vi "TabConAlt v0.1.vi"() -> ()   [LabVIEW 2017]
panel:
  out "strMAT":string
  in  "initMAT":bool
  out "statusMAT":bool
  out "connMAT":bool caption="Matisse TX"
  out "strMIL":string
  in  "initMIL":bool
  out "statusMIL":bool
  out "connMIL":bool caption="Millenia eV 25W"
  out "strCCD":string
  in  "initCCD":bool
  out "statusCCD":bool
  out "connCCD":bool caption="Pylon CCD"
  out "strSPT":string
  in  "initSPT":bool caption="Spectrometer"
  out "statusSPT":bool
  out "connSPT":bool caption="Spectrometer"
  out "strLIA":string
  in  "initLIA":bool caption="Lock-in"
  out "statusLIA":bool
  out "connLIA":bool caption="Lock-in & Chopper"
  in  "initALL":bool caption="Initialize all"
  in  "stopExecution":bool
  in  "clearNotifications":bool
  out "Notifications":string
  out "measRUN":bool caption="Measurement running"
  out "measREADY":bool caption="Measurement ready"
  out "UIbusy":bool caption="Interface busy"
  in  "Settings":T1(tab)
  in  "visaSPT":string caption="VISA address"
  in  "visaCCD":string caption="VISA address"
  in  "visaLIA":string caption="VISA address"
  in  "Chopping Frequency":dbl[unit](knob) scale=200.0..2000.0
  in  "Ring cavity  energy":cluster{dbl[unit], dbl[unit]}(slide) caption="Ring cavity  energy / eV"
  in  "Ring cavity wavelength":cluster{dbl[unit], dbl[unit]}(slide)={0.0, 9.616279069767442e-07} caption="Ring cavity wavelength / nm"
  in  "Enslave Millennia eV":bool
  in  "Installed Optics":string(combo)="MOS2 BB"
  in  "visaMAT":string caption="VISA address"
  in  "Matisse Power":dbl[unit](knob)=1e-06 caption="Millenia Power" min=1.0 max=25.0 scale=1.0..25.0
  in  "visaMIL":string caption="VISA address"
  in  "Millenia Power":dbl[unit](knob)=0.001 min=1.0 max=25.0 scale=1.0..25.0
  out "DummyVisaOut":string
  in  "mainqSize":dbl=1000.0 caption="Queue size" min=1.0 step=1.0
  in  "timebaseMaster":dbl[unit]=0.08 caption="Master timebase" min=0.0001 max=0.5 step=0.0001 format="%#_6f"
  in  "timebaseSlave":dbl[unit]=0.16 caption="Slave timebase" min=0.0001 max=0.5 step=0.0001
  in  "abbrSPT":string="SPT"
  in  "abbrCCD":string="CCD"
  in  "abbrMIL":string="MIL"
  in  "abbrMAT":string="MAT"
  in  "abbrLIA":string="LIA"
  in  "nameSPT":string="Spectrometer"
  in  "nameLIA":string="SRS865"
  in  "nameCCD":string="Pylon CCD"
  in  "nameMIL":string="Millennia eV 25W"
  in  "nameMAT":string="Matisse 2 TX"
  # "Lower"
  # "Upper"
  # "eV"
  # "eV"
  # "Lower"
  # "Upper"
  # "nm"
  # "nm"
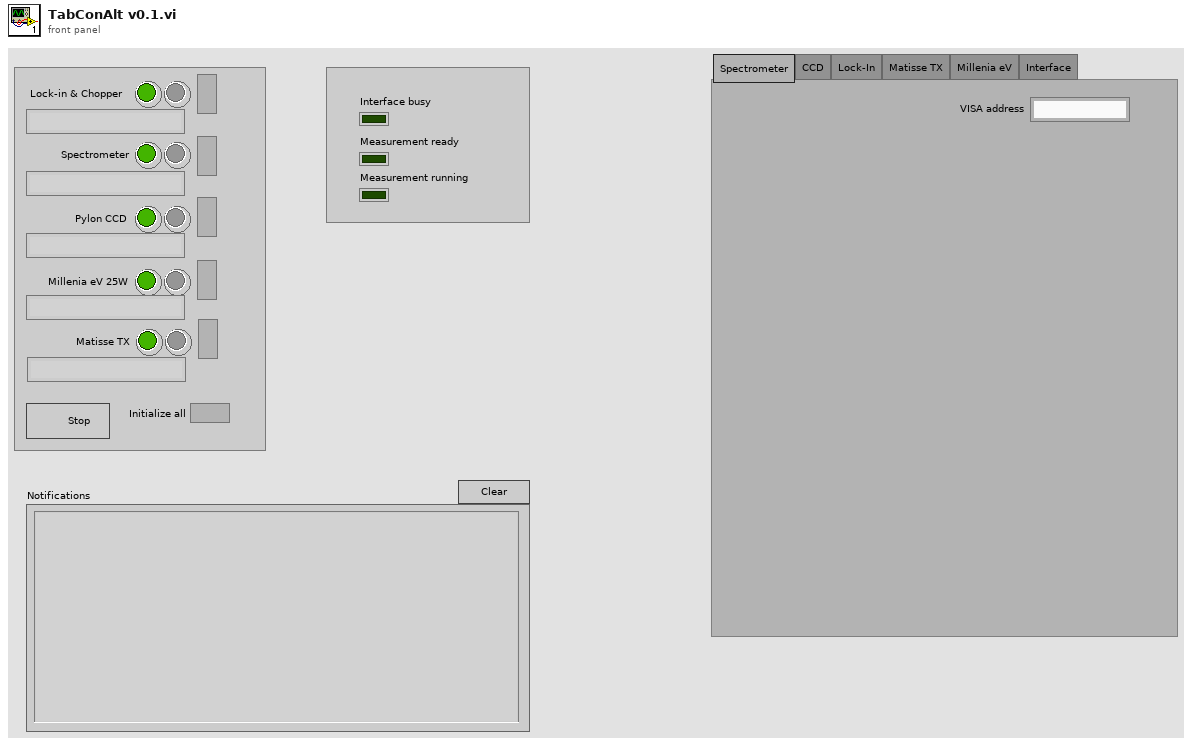
[diagram p1: front panel]
types:
  T1 = enum32{"Spectrometer", "CCD", "Lock-In", "Matisse TX", "Millenia eV", "Interface"}
  T2 = cluster{"elementArr":cluster{"cmd":string, "cmdclass":string, "data":variant}[]}
  T3 = cluster{"str":string, "ctlref":refnum<vi>, "newStatus":bool, "ctlstr":refnum<vi>}
  T4 = cluster{string, "chgStatusLED":refnum<user-event>}
  T5 = cluster{cluster{string, "chgStatusLED":refnum<user-event>}, cluster{string, "qintoMain":refnum<user-event>}}
  T6 = typedef "RefArray.ctl" = cluster{"String":string, "Array":refnum<vi>[]}[]
  T7 = cluster{"Command":string, "Command class":string, "Variant":variant}
  T8 = cluster{"Command":string, "Command class":string, "Variant":variant}[]
  T9 = cluster{"cmd":string, "cmdclass":string, "data":variant}[]
  T10 = typedef "eventsource.ctl" = u32
  T11 = cluster{"String":string, "String 2":string, "Variant":variant}[]
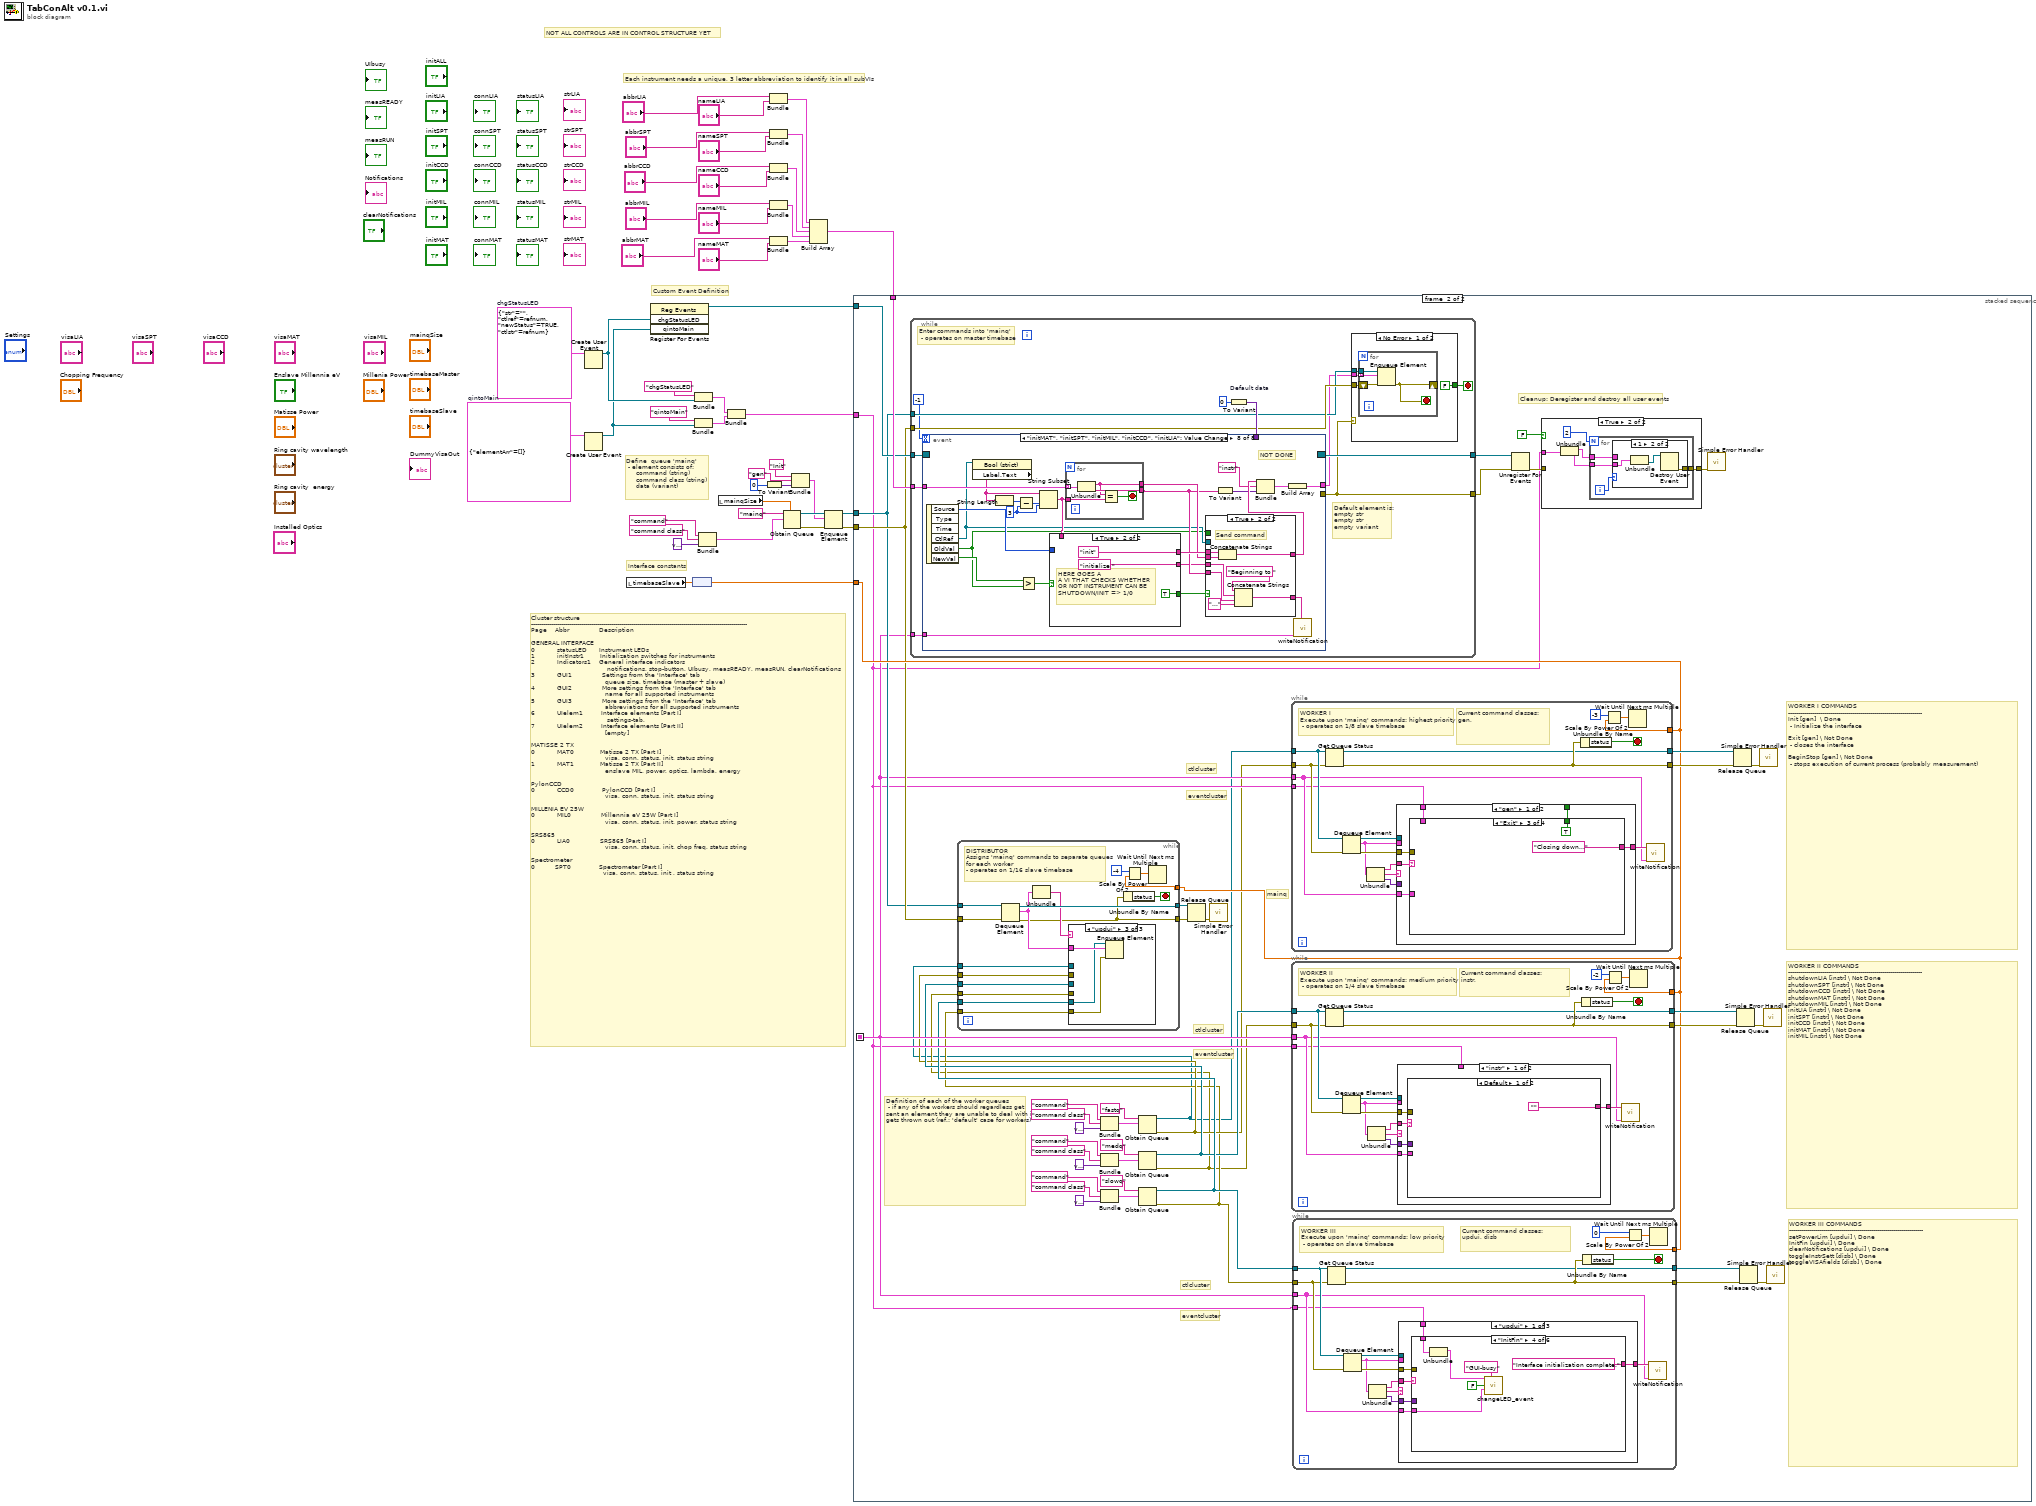
[diagram p0: block diagram]
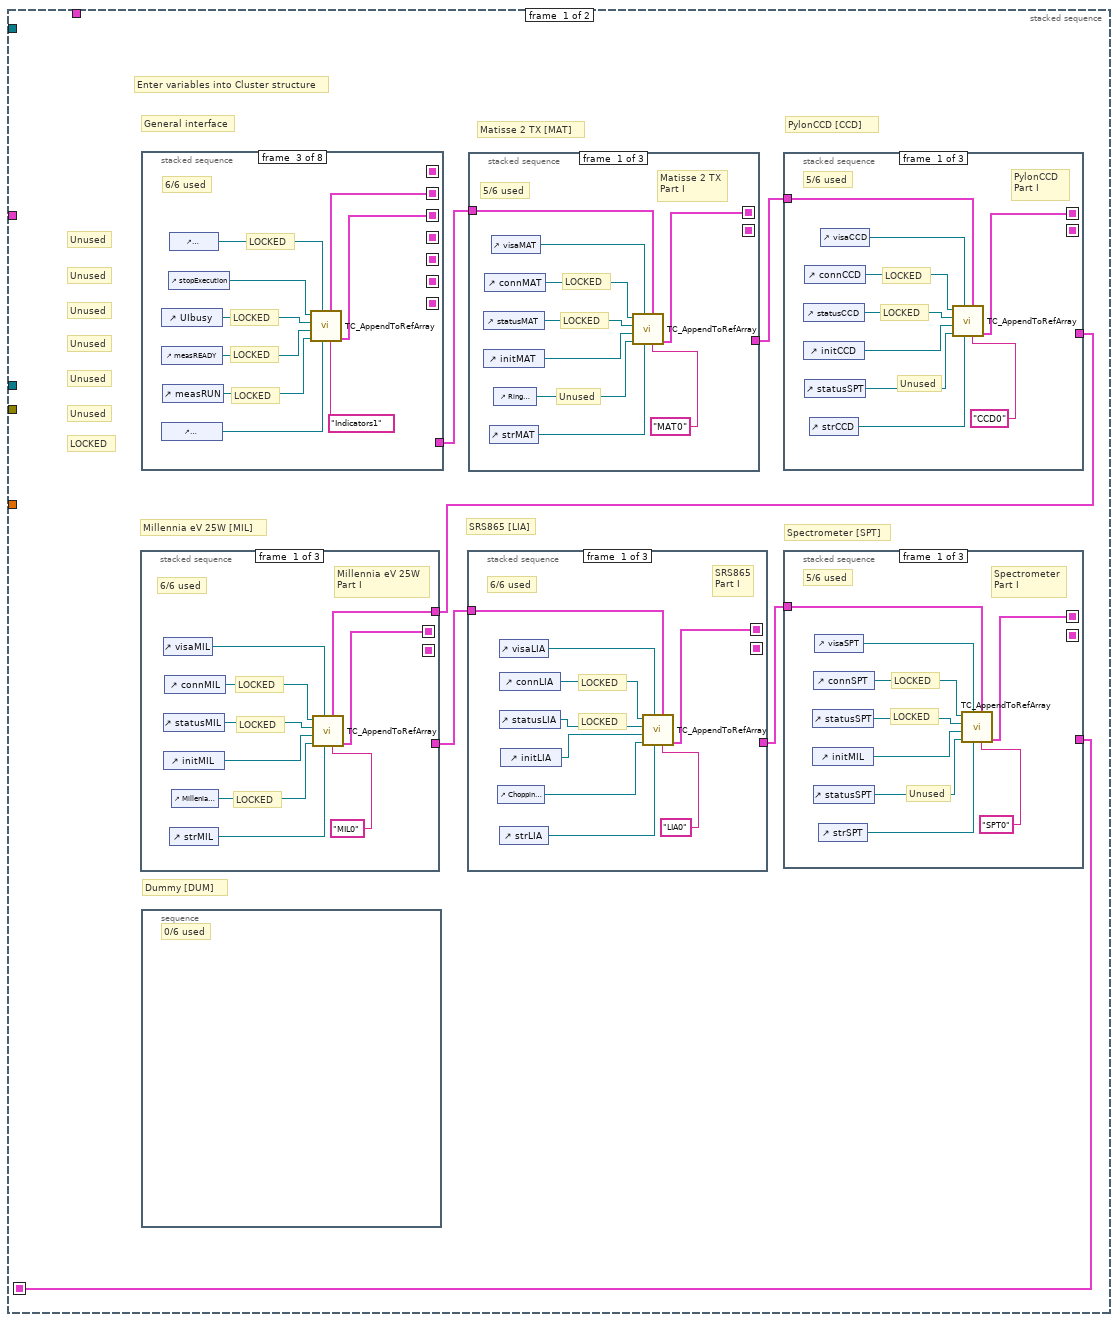
[diagram p2: hidden frame]
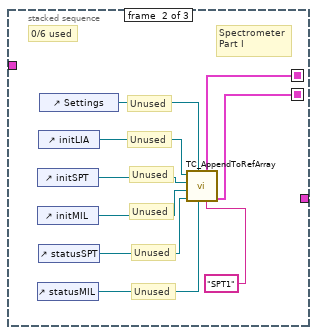
[diagram p3: hidden frame]
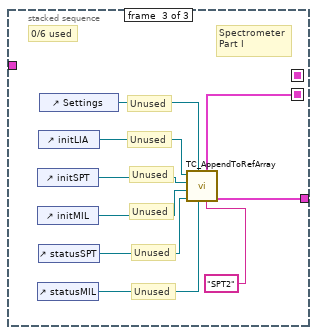
[diagram p4: hidden frame]
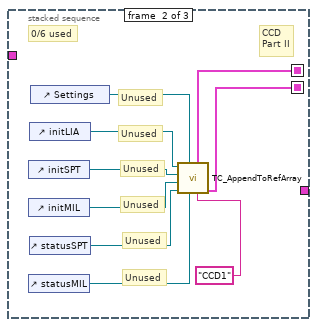
[diagram p5: hidden frame]
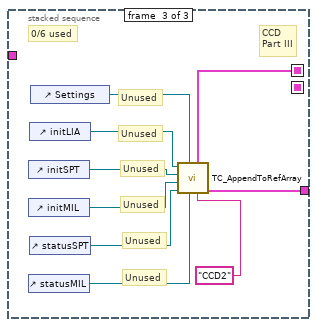
[diagram p6: hidden frame]
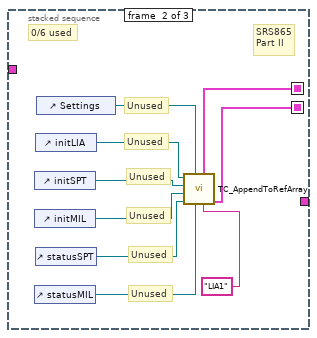
[diagram p7: hidden frame]
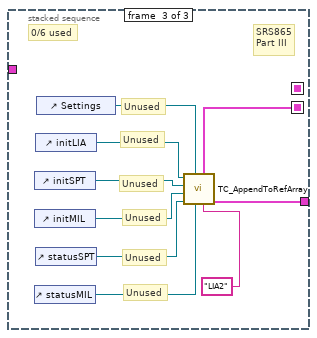
[diagram p8: hidden frame]
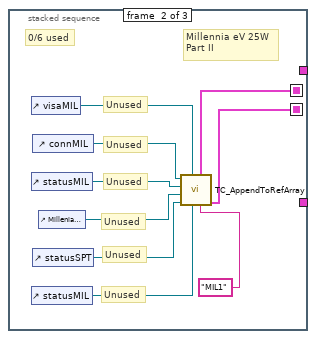
[diagram p9: hidden frame]
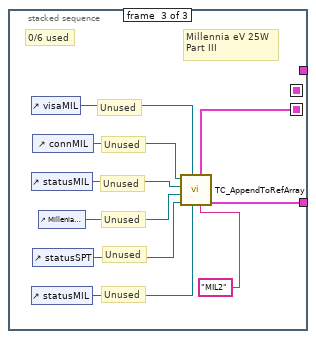
[diagram p10: hidden frame]
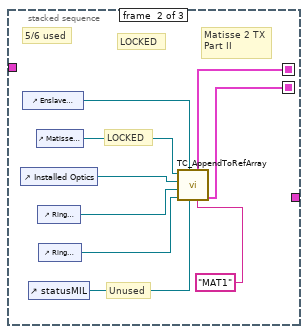
[diagram p11: hidden frame]
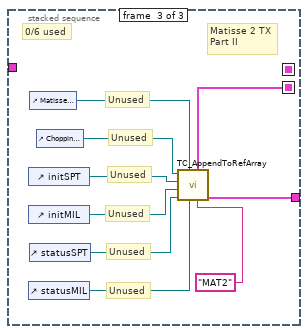
[diagram p12: hidden frame]
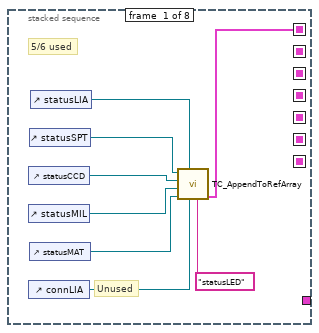
[diagram p13: hidden frame]
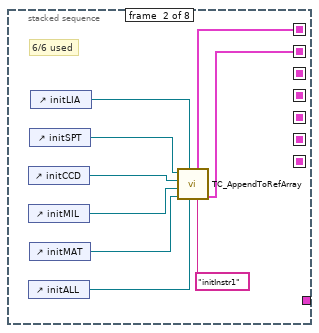
[diagram p14: hidden frame]
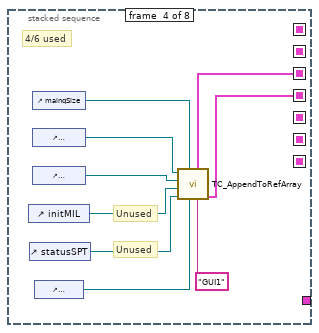
[diagram p15: hidden frame]
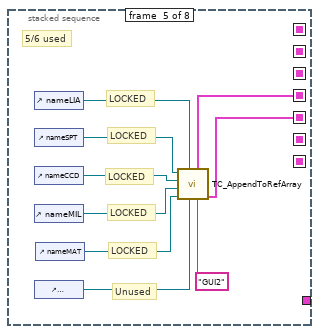
[diagram p16: hidden frame]
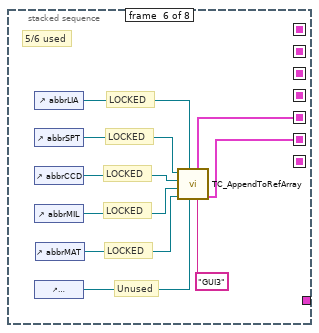
[diagram p17: hidden frame]
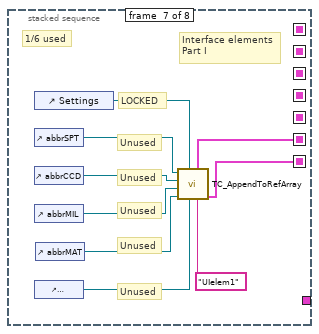
[diagram p18: hidden frame]
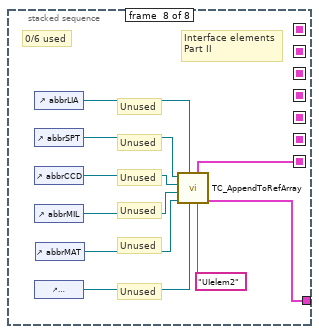
[diagram p19: hidden frame]
diagram:
  w13 = T2 {"elementArr"=[]}  # qintoMain
  w14 = T3 {"str"="", "ctlref"=refnum, "newStatus"=TRUE, "ctlstr"=refnum}  # chgStatusLED
  # "Custom Event Definition"
  # "Cluster structure\n------------------------------------------------------------------------------------------------------------\nPage    Abbr               Description\n\nGENERAL INTERFACE\n0           statusLED      Instrument LEDs\n1           initInstr1        Initialization switches for instruments\n2           Indicators1    General interface indicators\n                                      notifications, stop-button, UIbusy, measREADY, measRUN, clearNotifications\n3           GUI1               Settings from the 'Interface' tab\n                                     queue size, timebase (master + slave)\n4           GUI2               More settings from the 'Interface' tab\n                                     name for all supported instruments\n5           GUI3               More settings from the 'Interface' tab\n                                     abbreviations for all supported instruments\n6           UIelem1         Interface elements [Part I]\n                                      settings-tab,\n7           UIelem2         Interface elements [Part II]\n                                     [empty]\n\nMATISSE 2 TX\n0           MAT0             Matisse 2 TX [Part I]\n                                     visa, conn, status, init, status string\n1           MAT1             Matisse 2 TX [Part II]\n                                     enslave MIL, power, optics, lambda, energy\n\nPylonCCD\n0           CCD0              PylonCCD [Part I]\n                                     visa, conn, status, init, status string\n\nMILLENIA EV 25W\n0           MIL0               Millennia eV 25W [Part I]\n                                     visa, conn, status, init, power, status string\n\nSRS865\n0           LIA0               SRS865 [Part I]\n                                     visa, conn, status, init, chop freq, status string\n\nSpectrometer\n0          SPT0              Spectrometer [Part I]\n                                    visa, conn, status, init , status string"
  # "NOT ALL CONTROLS ARE IN CONTROL STRUCTURE YET"
  # "Each instrument needs a unique, 3 letter abbreviation to identify it in all subVIs"
  # "Define  queue 'mainq'\n - element consists of:\n     command (string)\n     command class (string)\n     data (variant)"
  # "Interface constants"
  n1 = Create User Event(user event datatype=w14) -> (user event=w12:refnum<user-event>)  [unwired: 1 in, 1 out]
  n2 = Create User Event(user event datatype=w13) -> (user event=w9:refnum<user-event>)  [unwired: 1 in, 1 out]
  n3 = local read "timebaseSlave"() -> (w33:dbl[unit])
  n4 = register-events(w12, w9) -> (reference out=w15:refnum<event-registration>)  [unwired: 2 in, 1 out]
  n5 = node(w33) -> (w32:dbl)
  n6 = Bundle("qintoMain", "qintoMain"=w9) -> (w2:cluster{string, "qintoMain":refnum<user-event>})  [unwired: 1 in]
  n7 = Bundle("chgStatusLED", "chgStatusLED"=w12) -> (w3:T4)  [unwired: 1 in]
  n8 = Bundle("command", "command class", variant) -> (w34:cluster{string, string, variant})  [unwired: 1 in]
  n9 = local read "mainqSize"() -> (w40:dbl)
  n10 = Bundle(w3, w2) -> (w1:T5)  [unwired: 1 in]
  n11 = To Variant(anything=0) -> (Variant=w42:variant)
  n12 = Bundle("abbrLIA"="abbrLIA", "nameLIA"="nameLIA") -> (w17:cluster{"abbrLIA":string, "nameLIA":string})  [unwired: 1 in]
  n13 = Bundle("abbrSPT"="abbrSPT", "nameSPT"="nameSPT") -> (w18:cluster{"abbrSPT":string, "nameSPT":string})  [unwired: 1 in]
  n14 = Bundle("abbrCCD"="abbrCCD", "nameCCD"="nameCCD") -> (w19:cluster{"abbrCCD":string, "nameCCD":string})  [unwired: 1 in]
  n15 = Bundle("abbrMIL"="abbrMIL", "nameMIL"="nameMIL") -> (w20:cluster{"abbrMIL":string, "nameMIL":string})  [unwired: 1 in]
  n16 = Bundle("abbrMAT"="abbrMAT", "nameMAT"="nameMAT") -> (w21:cluster{"abbrMAT":string, "nameMAT":string})  [unwired: 1 in]
  n17 = Obtain Queue(max queue size (-1, unlimited)=w40, name (unnamed)="mainq", element data type=w34) -> (queue out=w5:refnum<queue>, error out=w6:errorcluster)  [unwired: 2 in, 1 out]
  n18 = Bundle("Init", "gen", "Variant"=w42) -> (w4:cluster{string, string, "Variant":variant})  [unwired: 1 in]
  n19 = Build Array(w17, w18, w19, w20, w21) -> (w16:cluster{"abbrMAT":string, "nameMAT":string}[])
  n20 = Enqueue Element(queue=w5, element=w4, error in (no error)=w6) -> (queue out=w8:refnum<queue>, error out=w7:errorcluster)  [unwired: 1 in, 1 out]
  n21 = stacked-sequence {
    seq-local: [w44 _] -> [_ w263]
    tunnel: w32 -> [_ w275]
    tunnel: w16 -> [_ w273]
    tunnel: w15 -> [_ w269]
    tunnel: w1 -> [_ w262]
    tunnel: w8 -> [_ w264]
    tunnel: w7 -> [_ w265]
    frame #0 {
      # "LOCKED"
      # "Dummy [DUM]"
      # "Spectrometer [SPT]"
      # "PylonCCD [CCD]"
      # "Unused"
      # "Unused"
      # "Unused"
      # "Unused"
      # "Unused"
      # "Unused"
      # "SRS865 [LIA]"
      # "Millennia eV 25W [MIL]"
      # "General interface"
      # "Matisse 2 TX [MAT]"
      # "Enter variables into Cluster structure"
      n22 = stacked-sequence {
        seq-local: [w185 _ _ _ _ _ _ _] -> [_ w193 _ _ _ _ _ _]
        seq-local: [_ w194 _ _ _ _ _ _] -> [_ _ w204 _ _ _ _ _]
        seq-local: [_ _ w203 _ _ _ _ _] -> [_ _ _ w212 _ _ _ _]
        seq-local: [_ _ _ w211 _ _ _ _] -> [_ _ _ _ w221 _ _ _]
        seq-local: [_ _ _ _ w220 _ _ _] -> [_ _ _ _ _ w230 _ _]
        seq-local: [_ _ _ _ _ w229 _ _] -> [_ _ _ _ _ _ w239 _]
        seq-local: [_ _ _ _ _ _ w238 _] -> [_ _ _ _ _ _ _ w248]
        tunnel: [_ _ _ _ _ _ _ w247] -> w45
        frame #0 {
          # "Unused"
          # "5/6 used"
          n23 = control-ref of="statusCCD"() -> (w190:refnum<vi>)
          n24 = control-ref of="statusMIL"() -> (w189:refnum<vi>)
          n25 = control-ref of="connLIA"() -> (w187:refnum<vi>)
          n26 = control-ref of="statusSPT"() -> (w191:refnum<vi>)
          n27 = control-ref of="statusMAT"() -> (w188:refnum<vi>)
          n28 = control-ref of="statusLIA"() -> (w192:refnum<vi>)
          n29 = call "TC_AppendToRefArray.vi"("name"="statusLED", "ref6"=w187, "ref1"=w192, "ref5"=w188, "ref4"=w189, "ref3"=w190, "ref2"=w191) -> ("arrayOut"=w185:T6)  [unwired: 4 in]
        }
        frame #1 {
          # "6/6 used"
          n30 = control-ref of="initCCD"() -> (w199:refnum<vi>)
          n31 = control-ref of="initMIL"() -> (w198:refnum<vi>)
          n32 = control-ref of="initALL"() -> (w196:refnum<vi>)
          n33 = control-ref of="initSPT"() -> (w200:refnum<vi>)
          n34 = control-ref of="initMAT"() -> (w197:refnum<vi>)
          n35 = control-ref of="initLIA"() -> (w201:refnum<vi>)
          n36 = call "TC_AppendToRefArray.vi"("name"="initInstr1", "arrayIn"=w193, "ref6"=w196, "ref1"=w201, "ref5"=w197, "ref4"=w198, "ref3"=w199, "ref2"=w200) -> ("arrayOut"=w194:T6)  [unwired: 3 in]
        }
        frame #2 {
          # "LOCKED"
          # "LOCKED"
          # "LOCKED"
          # "LOCKED"
          # "6/6 used"
          n37 = control-ref of="UIbusy"() -> (w209:refnum<vi>)
          n38 = control-ref of="measREADY"() -> (w208:refnum<vi>)
          n39 = control-ref of="clearNotifications"() -> (w206:refnum<vi>)
          n40 = control-ref of="measRUN"() -> (w207:refnum<vi>)
          n41 = control-ref of="stopExecution"() -> (w202:refnum<vi>)
          n42 = control-ref of="Notifications"() -> (w210:refnum<vi>)
          n43 = call "TC_AppendToRefArray.vi"("name"="Indicators1", "arrayIn"=w204, "ref6"=w206, "ref1"=w210, "ref5"=w207, "ref4"=w208, "ref3"=w209, "ref2"=w202) -> ("arrayOut"=w203:T6)  [unwired: 3 in]
        }
        frame #3 {
          # "Unused"
          # "Unused"
          # "4/6 used"
          n44 = control-ref of="initMIL"() -> (w216:refnum<vi>)
          n45 = control-ref of="statusSPT"() -> (w215:refnum<vi>)
          n46 = control-ref of="mainqSize"() -> (w219:refnum<vi>)
          n47 = control-ref of="timebaseMaster"() -> (w218:refnum<vi>)
          n48 = control-ref of="timebaseSlave"() -> (w217:refnum<vi>)
          n49 = control-ref of="DummyVisaOut"() -> (w214:refnum<vi>)
          n50 = call "TC_AppendToRefArray.vi"("name"="GUI1", "arrayIn"=w212, "ref6"=w214, "ref1"=w219, "ref5"=w215, "ref4"=w216, "ref3"=w217, "ref2"=w218) -> ("arrayOut"=w211:T6)  [unwired: 3 in]
        }
        frame #4 {
          # "LOCKED"
          # "LOCKED"
          # "LOCKED"
          # "LOCKED"
          # "LOCKED"
          # "Unused"
          # "5/6 used"
          n51 = control-ref of="nameLIA"() -> (w228:refnum<vi>)
          n52 = control-ref of="nameSPT"() -> (w227:refnum<vi>)
          n53 = control-ref of="nameCCD"() -> (w226:refnum<vi>)
          n54 = control-ref of="nameMIL"() -> (w225:refnum<vi>)
          n55 = control-ref of="DummyVisaOut"() -> (w223:refnum<vi>)
          n56 = control-ref of="nameMAT"() -> (w224:refnum<vi>)
          n57 = call "TC_AppendToRefArray.vi"("name"="GUI2", "arrayIn"=w221, "ref6"=w223, "ref1"=w228, "ref5"=w224, "ref4"=w225, "ref3"=w226, "ref2"=w227) -> ("arrayOut"=w220:T6)  [unwired: 3 in]
        }
        frame #5 {
          # "LOCKED"
          # "LOCKED"
          # "LOCKED"
          # "LOCKED"
          # "LOCKED"
          # "Unused"
          # "5/6 used"
          n58 = control-ref of="abbrLIA"() -> (w237:refnum<vi>)
          n59 = control-ref of="abbrSPT"() -> (w236:refnum<vi>)
          n60 = control-ref of="abbrCCD"() -> (w235:refnum<vi>)
          n61 = control-ref of="abbrMIL"() -> (w234:refnum<vi>)
          n62 = control-ref of="DummyVisaOut"() -> (w232:refnum<vi>)
          n63 = control-ref of="abbrMAT"() -> (w233:refnum<vi>)
          n64 = call "TC_AppendToRefArray.vi"("name"="GUI3", "arrayIn"=w230, "ref6"=w232, "ref1"=w237, "ref5"=w233, "ref4"=w234, "ref3"=w235, "ref2"=w236) -> ("arrayOut"=w229:T6)  [unwired: 3 in]
        }
        frame #6 {
          # "LOCKED"
          # "Interface elements\nPart I"
          # "Unused"
          # "Unused"
          # "Unused"
          # "Unused"
          # "Unused"
          # "1/6 used"
          n65 = control-ref of="Settings"() -> (w246:refnum<vi>)
          n66 = control-ref of="abbrSPT"() -> (w245:refnum<vi>)
          n67 = control-ref of="abbrCCD"() -> (w244:refnum<vi>)
          n68 = control-ref of="abbrMIL"() -> (w243:refnum<vi>)
          n69 = control-ref of="DummyVisaOut"() -> (w241:refnum<vi>)
          n70 = control-ref of="abbrMAT"() -> (w242:refnum<vi>)
          n71 = call "TC_AppendToRefArray.vi"("name"="UIelem1", "arrayIn"=w239, "ref6"=w241, "ref1"=w246, "ref5"=w242, "ref4"=w243, "ref3"=w244, "ref2"=w245) -> ("arrayOut"=w238:T6)  [unwired: 3 in]
        }
        frame #7 {
          # "Interface elements\nPart II"
          # "Unused"
          # "Unused"
          # "Unused"
          # "Unused"
          # "Unused"
          # "Unused"
          # "0/6 used"
          n72 = control-ref of="abbrLIA"() -> (w255:refnum<vi>)
          n73 = control-ref of="abbrSPT"() -> (w254:refnum<vi>)
          n74 = control-ref of="abbrCCD"() -> (w253:refnum<vi>)
          n75 = control-ref of="abbrMIL"() -> (w252:refnum<vi>)
          n76 = control-ref of="DummyVisaOut"() -> (w250:refnum<vi>)
          n77 = control-ref of="abbrMAT"() -> (w251:refnum<vi>)
          n78 = call "TC_AppendToRefArray.vi"("name"="UIelem2", "arrayIn"=w248, "ref6"=w250, "ref1"=w255, "ref5"=w251, "ref4"=w252, "ref3"=w253, "ref2"=w254) -> ("arrayOut"=w247:T6)  [unwired: 3 in]
        }
      }
      n79 = stacked-sequence {
        frame #0 {
          # "0/6 used"
        }
      }
      n80 = stacked-sequence {
        seq-local: [w158 _ _] -> [_ w168 _]
        seq-local: [_ w167 _] -> [_ _ w176]
        tunnel: w45 -> [w159 _ _]
        tunnel: [_ _ w177] -> w47
        frame #0 {
          # "LOCKED"
          # "LOCKED"
          # "Unused"
          # "Matisse 2 TX\nPart I"
          # "5/6 used"
          n81 = control-ref of="statusMAT"() -> (w163:refnum<vi>)
          n82 = control-ref of="initMAT"() -> (w164:refnum<vi>)
          n83 = control-ref of="connMAT"() -> (w162:refnum<vi>)
          n84 = control-ref of="strMAT"() -> (w166:refnum<vi>)
          n85 = control-ref of="visaMAT"() -> (w161:refnum<vi>)
          n86 = control-ref of="Ring cavity  energy"() -> (w165:refnum<vi>)
          n87 = call "TC_AppendToRefArray.vi"("name"="MAT0", "arrayIn"=w159, "ref6"=w166, "ref1"=w161, "ref5"=w165, "ref4"=w164, "ref3"=w163, "ref2"=w162) -> ("arrayOut"=w158:T6)  [unwired: 3 in]
        }
        frame #1 {
          # "LOCKED"
          # "LOCKED"
          # "Unused"
          # "Matisse 2 TX\nPart II"
          # "5/6 used"
          n88 = control-ref of="Installed Optics"() -> (w172:refnum<vi>)
          n89 = control-ref of="Enslave Millennia eV"() -> (w170:refnum<vi>)
          n90 = control-ref of="statusMIL"() -> (w175:refnum<vi>)
          n91 = control-ref of="Matisse Power"() -> (w171:refnum<vi>)
          n92 = control-ref of="Ring cavity wavelength"() -> (w173:refnum<vi>)
          n93 = control-ref of="Ring cavity  energy"() -> (w174:refnum<vi>)
          n94 = call "TC_AppendToRefArray.vi"("name"="MAT1", "arrayIn"=w168, "ref6"=w175, "ref1"=w170, "ref5"=w174, "ref4"=w173, "ref3"=w172, "ref2"=w171) -> ("arrayOut"=w167:T6)  [unwired: 3 in]
        }
        frame #2 {
          # "Unused"
          # "Unused"
          # "Unused"
          # "Unused"
          # "Unused"
          # "Unused"
          # "Matisse 2 TX\nPart II"
          # "0/6 used"
          n95 = control-ref of="initSPT"() -> (w181:refnum<vi>)
          n96 = control-ref of="initMIL"() -> (w182:refnum<vi>)
          n97 = control-ref of="statusMIL"() -> (w184:refnum<vi>)
          n98 = control-ref of="Matisse Power"() -> (w179:refnum<vi>)
          n99 = control-ref of="statusSPT"() -> (w183:refnum<vi>)
          n100 = control-ref of="Chopping Frequency"() -> (w180:refnum<vi>)
          n101 = call "TC_AppendToRefArray.vi"("name"="MAT2", "arrayIn"=w176, "ref6"=w184, "ref1"=w179, "ref5"=w183, "ref4"=w182, "ref3"=w181, "ref2"=w180) -> ("arrayOut"=w177:T6)  [unwired: 3 in]
        }
      }
      n102 = stacked-sequence {
        seq-local: [w77 _ _] -> [_ w87 w96]
        seq-local: [_ w86 _] -> [_ _ _]
        tunnel: w47 -> [w78 _ _]
        tunnel: [_ _ w95] -> w48
        frame #0 {
          # "LOCKED"
          # "LOCKED"
          # "PylonCCD\nPart I"
          # "Unused"
          # "5/6 used"
          n103 = control-ref of="statusCCD"() -> (w82:refnum<vi>)
          n104 = control-ref of="initCCD"() -> (w83:refnum<vi>)
          n105 = control-ref of="connCCD"() -> (w81:refnum<vi>)
          n106 = control-ref of="statusSPT"() -> (w84:refnum<vi>)
          n107 = control-ref of="strCCD"() -> (w85:refnum<vi>)
          n108 = control-ref of="visaCCD"() -> (w80:refnum<vi>)
          n109 = call "TC_AppendToRefArray.vi"("name"="CCD0", "arrayIn"=w78, "ref6"=w85, "ref1"=w80, "ref5"=w84, "ref4"=w83, "ref3"=w82, "ref2"=w81) -> ("arrayOut"=w77:T6)  [unwired: 3 in]
        }
        frame #1 {
          # "CCD\nPart II"
          # "Unused"
          # "Unused"
          # "Unused"
          # "Unused"
          # "Unused"
          # "Unused"
          # "0/6 used"
          n110 = control-ref of="initSPT"() -> (w91:refnum<vi>)
          n111 = control-ref of="initMIL"() -> (w92:refnum<vi>)
          n112 = control-ref of="statusMIL"() -> (w94:refnum<vi>)
          n113 = control-ref of="initLIA"() -> (w90:refnum<vi>)
          n114 = control-ref of="statusSPT"() -> (w93:refnum<vi>)
          n115 = control-ref of="Settings"() -> (w89:refnum<vi>)
          n116 = call "TC_AppendToRefArray.vi"("name"="CCD1", "arrayIn"=w87, "ref6"=w94, "ref1"=w89, "ref5"=w93, "ref4"=w92, "ref3"=w91, "ref2"=w90) -> ("arrayOut"=w86:T6)  [unwired: 3 in]
        }
        frame #2 {
          # "CCD\nPart III"
          # "Unused"
          # "Unused"
          # "Unused"
          # "Unused"
          # "Unused"
          # "Unused"
          # "0/6 used"
          n117 = control-ref of="initSPT"() -> (w100:refnum<vi>)
          n118 = control-ref of="initMIL"() -> (w101:refnum<vi>)
          n119 = control-ref of="statusMIL"() -> (w103:refnum<vi>)
          n120 = control-ref of="initLIA"() -> (w99:refnum<vi>)
          n121 = control-ref of="statusSPT"() -> (w102:refnum<vi>)
          n122 = control-ref of="Settings"() -> (w98:refnum<vi>)
          n123 = call "TC_AppendToRefArray.vi"("name"="CCD2", "arrayIn"=w96, "ref6"=w103, "ref1"=w98, "ref5"=w102, "ref4"=w101, "ref3"=w100, "ref2"=w99) -> ("arrayOut"=w95:T6)  [unwired: 3 in]
        }
      }
      n124 = stacked-sequence {
        seq-local: [w131 _ _] -> [_ w141 _]
        seq-local: [_ w140 _] -> [_ _ w150]
        tunnel: w48 -> [w132 _ _]
        tunnel: [_ _ w149] -> w46
        frame #0 {
          # "LOCKED"
          # "LOCKED"
          # "LOCKED"
          # "Millennia eV 25W\nPart I"
          # "6/6 used"
          n125 = control-ref of="visaMIL"() -> (w134:refnum<vi>)
          n126 = control-ref of="statusMIL"() -> (w136:refnum<vi>)
          n127 = control-ref of="initMIL"() -> (w137:refnum<vi>)
          n128 = control-ref of="connMIL"() -> (w135:refnum<vi>)
          n129 = control-ref of="strMIL"() -> (w139:refnum<vi>)
          n130 = control-ref of="Millenia Power"() -> (w138:refnum<vi>)
          n131 = call "TC_AppendToRefArray.vi"("name"="MIL0", "arrayIn"=w132, "ref6"=w139, "ref1"=w134, "ref5"=w138, "ref4"=w137, "ref3"=w136, "ref2"=w135) -> ("arrayOut"=w131:T6)  [unwired: 3 in]
        }
        frame #1 {
          # "Unused"
          # "Unused"
          # "Unused"
          # "Unused"
          # "Unused"
          # "Unused"
          # "Millennia eV 25W\nPart II"
          # "0/6 used"
          n132 = control-ref of="visaMIL"() -> (w143:refnum<vi>)
          n133 = control-ref of="statusMIL"() -> (w145:refnum<vi>)
          n134 = control-ref of="statusMIL"() -> (w148:refnum<vi>)
          n135 = control-ref of="connMIL"() -> (w144:refnum<vi>)
          n136 = control-ref of="statusSPT"() -> (w147:refnum<vi>)
          n137 = control-ref of="Millenia Power"() -> (w146:refnum<vi>)
          n138 = call "TC_AppendToRefArray.vi"("name"="MIL1", "arrayIn"=w141, "ref6"=w148, "ref1"=w143, "ref5"=w147, "ref4"=w146, "ref3"=w145, "ref2"=w144) -> ("arrayOut"=w140:T6)  [unwired: 3 in]
        }
        frame #2 {
          # "Unused"
          # "Unused"
          # "Unused"
          # "Unused"
          # "Unused"
          # "Unused"
          # "Millennia eV 25W\nPart III"
          # "0/6 used"
          n139 = control-ref of="visaMIL"() -> (w152:refnum<vi>)
          n140 = control-ref of="statusMIL"() -> (w154:refnum<vi>)
          n141 = control-ref of="statusMIL"() -> (w157:refnum<vi>)
          n142 = control-ref of="connMIL"() -> (w153:refnum<vi>)
          n143 = control-ref of="statusSPT"() -> (w156:refnum<vi>)
          n144 = control-ref of="Millenia Power"() -> (w155:refnum<vi>)
          n145 = call "TC_AppendToRefArray.vi"("name"="MIL2", "arrayIn"=w150, "ref6"=w157, "ref1"=w152, "ref5"=w156, "ref4"=w155, "ref3"=w154, "ref2"=w153) -> ("arrayOut"=w149:T6)  [unwired: 3 in]
        }
      }
      n146 = stacked-sequence {
        seq-local: [w108 _ _] -> [_ w114 _]
        seq-local: [_ w113 _] -> [_ _ w122]
        tunnel: w46 -> [w109 _ _]
        tunnel: [_ _ w123] -> w49
        frame #0 {
          # "LOCKED"
          # "LOCKED"
          # "SRS865\nPart I"
          # "6/6 used"
          n147 = control-ref of="Chopping Frequency"() -> (w107:refnum<vi>)
          n148 = control-ref of="visaLIA"() -> (w111:refnum<vi>)
          n149 = control-ref of="connLIA"() -> (w104:refnum<vi>)
          n150 = control-ref of="statusLIA"() -> (w105:refnum<vi>)
          n151 = control-ref of="strLIA"() -> (w112:refnum<vi>)
          n152 = control-ref of="initLIA"() -> (w106:refnum<vi>)
          n153 = call "TC_AppendToRefArray.vi"("name"="LIA0", "arrayIn"=w109, "ref6"=w112, "ref1"=w111, "ref5"=w107, "ref4"=w106, "ref3"=w105, "ref2"=w104) -> ("arrayOut"=w108:T6)  [unwired: 3 in]
        }
        frame #1 {
          # "Unused"
          # "Unused"
          # "Unused"
          # "Unused"
          # "Unused"
          # "Unused"
          # "SRS865\nPart II"
          # "0/6 used"
          n154 = control-ref of="initSPT"() -> (w118:refnum<vi>)
          n155 = control-ref of="initMIL"() -> (w119:refnum<vi>)
          n156 = control-ref of="statusMIL"() -> (w121:refnum<vi>)
          n157 = control-ref of="initLIA"() -> (w117:refnum<vi>)
          n158 = control-ref of="statusSPT"() -> (w120:refnum<vi>)
          n159 = control-ref of="Settings"() -> (w116:refnum<vi>)
          n160 = call "TC_AppendToRefArray.vi"("name"="LIA1", "arrayIn"=w114, "ref6"=w121, "ref1"=w116, "ref5"=w120, "ref4"=w119, "ref3"=w118, "ref2"=w117) -> ("arrayOut"=w113:T6)  [unwired: 3 in]
        }
        frame #2 {
          # "Unused"
          # "Unused"
          # "Unused"
          # "Unused"
          # "Unused"
          # "Unused"
          # "SRS865\nPart III"
          # "0/6 used"
          n161 = control-ref of="initSPT"() -> (w127:refnum<vi>)
          n162 = control-ref of="initMIL"() -> (w128:refnum<vi>)
          n163 = control-ref of="statusMIL"() -> (w130:refnum<vi>)
          n164 = control-ref of="initLIA"() -> (w126:refnum<vi>)
          n165 = control-ref of="statusSPT"() -> (w129:refnum<vi>)
          n166 = control-ref of="Settings"() -> (w125:refnum<vi>)
          n167 = call "TC_AppendToRefArray.vi"("name"="LIA2", "arrayIn"=w122, "ref6"=w130, "ref1"=w125, "ref5"=w129, "ref4"=w128, "ref3"=w127, "ref2"=w126) -> ("arrayOut"=w123:T6)  [unwired: 3 in]
        }
      }
      n168 = stacked-sequence {
        seq-local: [w50 _ _] -> [_ w60 _]
        seq-local: [_ w59 _] -> [_ _ w69]
        tunnel: w49 -> [w51 _ _]
        tunnel: [_ _ w68] -> w44
        frame #0 {
          # "LOCKED"
          # "LOCKED"
          # "Spectrometer\nPart I"
          # "Unused"
          # "5/6 used"
          n169 = control-ref of="statusSPT"() -> (w55:refnum<vi>)
          n170 = control-ref of="initMIL"() -> (w56:refnum<vi>)
          n171 = control-ref of="connSPT"() -> (w54:refnum<vi>)
          n172 = control-ref of="statusSPT"() -> (w57:refnum<vi>)
          n173 = control-ref of="visaSPT"() -> (w53:refnum<vi>)
          n174 = control-ref of="strSPT"() -> (w58:refnum<vi>)
          n175 = call "TC_AppendToRefArray.vi"("name"="SPT0", "arrayIn"=w51, "ref6"=w58, "ref1"=w53, "ref5"=w57, "ref4"=w56, "ref3"=w55, "ref2"=w54) -> ("arrayOut"=w50:T6)  [unwired: 3 in]
        }
        frame #1 {
          # "Spectrometer\nPart I"
          # "Unused"
          # "Unused"
          # "Unused"
          # "Unused"
          # "Unused"
          # "Unused"
          # "0/6 used"
          n176 = control-ref of="initSPT"() -> (w64:refnum<vi>)
          n177 = control-ref of="initMIL"() -> (w65:refnum<vi>)
          n178 = control-ref of="statusMIL"() -> (w67:refnum<vi>)
          n179 = control-ref of="initLIA"() -> (w63:refnum<vi>)
          n180 = control-ref of="statusSPT"() -> (w66:refnum<vi>)
          n181 = control-ref of="Settings"() -> (w62:refnum<vi>)
          n182 = call "TC_AppendToRefArray.vi"("name"="SPT1", "arrayIn"=w60, "ref6"=w67, "ref1"=w62, "ref5"=w66, "ref4"=w65, "ref3"=w64, "ref2"=w63) -> ("arrayOut"=w59:T6)  [unwired: 3 in]
        }
        frame #2 {
          # "Spectrometer\nPart I"
          # "Unused"
          # "Unused"
          # "Unused"
          # "Unused"
          # "Unused"
          # "Unused"
          # "0/6 used"
          n183 = control-ref of="initSPT"() -> (w73:refnum<vi>)
          n184 = control-ref of="initMIL"() -> (w74:refnum<vi>)
          n185 = control-ref of="statusMIL"() -> (w76:refnum<vi>)
          n186 = control-ref of="initLIA"() -> (w72:refnum<vi>)
          n187 = control-ref of="statusSPT"() -> (w75:refnum<vi>)
          n188 = control-ref of="Settings"() -> (w71:refnum<vi>)
          n189 = call "TC_AppendToRefArray.vi"("name"="SPT2", "arrayIn"=w69, "ref6"=w76, "ref1"=w71, "ref5"=w75, "ref4"=w74, "ref3"=w73, "ref2"=w72) -> ("arrayOut"=w68:T6)  [unwired: 3 in]
        }
      }
    }
    frame #1 {
      # "Cleanup: Deregister and destroy all user events"
      # "ctlcluster"
      # "eventcluster"
      # "ctlcluster"
      # "eventcluster"
      # "ctlcluster"
      # "eventcluster"
      # "WORKER III COMMANDS\n-------------------------------------------------------------------\nsetPowerLim [updui] \\ Done\nInitFin [updui] \\ Done\nclearNotifications [updui] \\ Done\ntoggleInstrSett [disb] \\ Done \ntoggleVISAfields [disb] \\ Done"
      # "WORKER II COMMANDS\n-------------------------------------------------------------------\nshutdownLIA [instr] \\ Not Done\nshutdownSPT [instr] \\ Not Done\nshutdownCCD [instr] \\ Not Done\nshutdownMAT [instr] \\ Not Done\nshutdownMIL [instr] \\ Not Done\ninitLIA [instr] \\ Not Done\ninitSPT [instr] \\ Not Done\ninitCCD [instr] \\ Not Done\ninitMAT [instr] \\ Not Done\ninitMIL [instr] \\ Not Done"
      # "WORKER I COMMANDS\n-------------------------------------------------------------------\nInit [gen]  \\ Done\n - Initialize the interface\n\nExit [gen] \\ Not Done\n - closes the interface\n\nBeginStop [gen] \\ Not Done\n - stops execution of current process (probably measurement)"
      # "mainq"
      # "Definition of each of the worker queues\n - if any of the workers should regardless get   sent an element they are unable to deal with it gets thrown out (ref.: 'default' case for workers)"
      n190 = while {
        tunnel: w264 -> [w467]
        tunnel: w265 -> [w468]
        tunnel: w273 -> [w464]
        tunnel: w263 -> [w463]
        tunnel: [w461] -> w270
        tunnel: w269 -> [w470]
        tunnel: [w469] -> w297
        stop <- w466 stop-if-true
        # "Default element is:\nempty str\nempty str\nempty variant"
        # "Enter commands into 'mainq'\n - operates on master timebase"
        n191 = To Variant "Default data"(anything=0) -> (Variant=w472:variant)
        n192 = event shown="[7] \"initMAT\", \"initSPT\", \"initMIL\", \"initCCD\", \"initLIA\": Value Change" {
          selector: w470 -> [_ _ _ _ _ _ _ _]
          dyn-events: [_ _ _ _ _ _ _ _] -> w469
          timeout: -1 -> [_ _ _ _ _ _ _ _]
          tunnel: w472 -> [_ w492 w495 _ w509 _ _ _]
          tunnel: [_ w493 w498 _ w510 _ w540 w549] -> w465
          tunnel: w464 -> [_ _ _ _ _ _ _ w562]
          tunnel: w463 -> [_ _ _ _ _ _ _ w551]
          tunnel: [_ _ _ _ _ w519 _ _] -> w461
          event Timeout {
            n193 = event-data() -> ()  [unwired: 1 in, 3 out]
          }
          event "stopExecution": Value Change {
            w490 = "gen"  # Command class
            w489 = "BeginStop"  # Command
            n194 = event-data() -> ()  [unwired: 1 in, 3 out]
            n195 = Bundle("Command"=w489, "Command class"=w490, "Variant"=w492) -> (w491:T7)  [unwired: 1 in]
            n196 = Build Array(w491) -> (w493:T8)
          }
          event Panel Close? {
            w496 = "gen"  # Command class
            w497 = "Exit"  # Command
            n197 = event-data() -> ()  [unwired: 1 in, 4 out]
            n198 = Bundle("Command"=w497, "Command class"=w496, "Variant"=w495) -> (w494:T7)  [unwired: 1 in]
            n199 = event-data() -> ()  [unwired: 2 in, 1 out]
            n200 = Build Array(w494) -> (w498:T8)
          }
          event User Event {
            n201 = event-data() -> ("str"=w499:string, "ctlref"=w504:refnum<vi>, "newStatus"=w503:bool, "ctlstr"=w500:refnum<vi>)  [unwired: 1 in, 4 out]
            n202 = Not Equal?(x="default", y=w499) -> (x != y?=w501:bool)
            n203 = property on="Property Node" class="Bool (strict)"(reference=w504, "Val(Sgnl)"=w503) -> ()  [unwired: 1 in, 2 out]
            n204 = case shown="False" w501 {
              tunnel: w500 -> [_ w506]
              tunnel: w499 -> [_ w505]
              frame False {
              }
              frame True {
                n205 = property on="Property Node" class="Str"(reference=w506, "Val(Sgnl)"=w505) -> ()  [unwired: 1 in, 2 out]
              }
            }
          }
          event "clearNotifications": Value Change {
            n206 = event-data() -> ("OldVal"=w514:bool, "NewVal"=w513:bool)  [unwired: 1 in, 4 out]
            n207 = Less?(x=w514, y=w513) -> (x < y?=w512:bool)
            n208 = case shown="True" w512 {
              tunnel: ["" "clearNotifications"] -> w508
              tunnel: ["gen" "updui"] -> w507
              frame False {
              }
              frame True {
              }
            }
            n209 = Bundle(w508, w507, "Variant"=w509) -> (w511:cluster{string, string, "Variant":variant})  [unwired: 1 in]
            n210 = Build Array(w511) -> (w510:cluster{string, string, "Variant":variant}[])
          }
          event "initALL": Value Change {
            n211 = event-data() -> ("OldVal"=w525:bool, "NewVal"=w524:bool)  [unwired: 1 in, 4 out]
            n212 = control-ref of="initMAT"() -> (w521:refnum<vi>)
            n213 = control-ref of="initCCD"() -> (w522:refnum<vi>)
            n214 = control-ref of="initMIL"() -> (w527:refnum<vi>)
            n215 = control-ref of="initLIA"() -> (w529:refnum<vi>)
            n216 = control-ref of="initSPT"() -> (w528:refnum<vi>)
            n217 = Build Array(w529, w528, w527, w522, w521) -> (w526:refnum<vi>[])
            n218 = Less?(x=w525, y=w524) -> (x < y?=w523:bool)
            n219 = case shown="False" w523 {
              selector: w523 -> [_ w539]
              tunnel: [w537 w539] -> w520
              frame False {
                n220 = Two Button Dialog(message="Disconnect all instruments?") -> (T button?=w537:bool)  [unwired: 2 in]
              }
              frame True {
              }
            }
            n221 = case shown="True" w520 {
              tunnel: w526 -> [_ w532]
              tunnel: w524 -> [_ w531]
              tunnel: [_ w530] -> w519
              frame False {
              }
              frame True {
                n222 = for {
                  tunnel: w532 -> [w536] mode=indexing
                  shift-right: [w535] -> w530
                  shift-left: _ -> [w534]
                  tunnel: w531 -> [w533]
                  n223 = property class="Bool (strict)"(reference=w536, error in=w534, "Val(Sgnl)"=w533) -> (error out=w535:errorcluster)  [unwired: 1 out]
                }
              }
            }
          }
          event User Event {
            n224 = event-data() -> ("elementArr"=w540:T9)  [unwired: 1 in, 4 out]
          }
          event "initMAT", "initSPT", "initMIL", "initCCD", "initLIA": Value Change {
            w559 = 3
            # "NOT DONE"
            n225 = event-data() -> ("Source"=w563:T10, "CtlRef"=w542:refnum<vi>, "OldVal"=w541:bool, "NewVal"=w556:bool)  [unwired: 1 in, 2 out]
            n226 = property class="Bool (strict)"(reference=w542) -> ("Label.Text"=w560:string)  [unwired: 1 in, 2 out]
            n227 = String Length(string=w560) -> (length=w561:i32)
            n228 = Subtract(x=w561, y=w559) -> (x-y=w558:i32)
            n229 = Greater?(x=w556, y=w541) -> (0:w557:bool)
            n230 = String Subset(string=w560, offset (0)=w558, length (rest)=w559) -> (substring=w555:string)
            n231 = case shown="True" w557 {
              tunnel: w563 -> [_ _]
              tunnel: ["shutdown" "init"] -> w553
              tunnel: w555 -> [_ _]
              tunnel: [TRUE TRUE] -> w554
              tunnel: ["shut down " "initialize "] -> w544
              frame False {
                # "HERE GOES A\nA VI THAT CHECKS WHETHER\nOR NOT INSTRUMENT CAN BE \nSHUTDOWN/INIT => 1/0"
              }
              frame True {
                # "HERE GOES A\nA VI THAT CHECKS WHETHER\nOR NOT INSTRUMENT CAN BE \nSHUTDOWN/INIT => 1/0"
              }
            }
            n232 = for {
              tunnel: w562 -> [w584] mode=indexing
              tunnel: w555 -> [w583]
              tunnel: [w581] -> w545
              tunnel: [w580] -> w552
              stop <- w582 stop-if-true
              n233 = Unbundle(w584) -> ("abbrMAT"=w580:string, "nameMAT"=w581:string)
              n234 = Equal?(x=w580, y=w583) -> (x = y?=w582:bool)
            }
            n235 = case shown="True" w554 {
              tunnel: w553 -> [_ w579]
              tunnel: w552 -> [_ w578]
              tunnel: ["" w577] -> w548
              tunnel: w545 -> [w566 w576]
              tunnel: w544 -> [w567 w574]
              tunnel: [w570 w572] -> w543
              tunnel: w542 -> [w565 _]
              tunnel: w541 -> [w564 _]
              frame False {
                # "Don't send command."
                n236 = property class="Bool (strict)"(reference=w565, "Value"=w564) -> ()  [unwired: 1 in, 2 out]
                n237 = Concatenate Strings("Unable to ", w567, w566, ".") -> (w570:string)
              }
              frame True {
                # "Send command"
                n238 = Concatenate Strings(w579, w578) -> (w577:string)
                n239 = Concatenate Strings("Beginning to ", w574, w576, "...") -> (w572:string)
              }
            }
            n240 = To Variant(anything=w545) -> (Variant=w546:variant)
            n241 = Bundle(w548, "instr", "Variant"=w546) -> (w550:cluster{string, string, "Variant":variant})  [unwired: 1 in]
            n242 = Build Array(w550) -> (w549:cluster{string, string, "Variant":variant}[])
            n243 = call "writeNotification.vi"("string"=w543, "Array"=w551) -> ()  [unwired: 10 in]
          }
        }
        n244 = case shown="No Error" w461 {
          tunnel: w468 -> [w476 w486]
          tunnel: w467 -> [w475 w487]
          tunnel: [FALSE TRUE] -> w466
          tunnel: w465 -> [w474 _]
          frame No Error {
            n245 = for {
              tunnel: w474 -> [w479] mode=indexing
              tunnel: w475 -> [w478]
              shift-right: [w477] -> _
              shift-left: w476 -> [w480]
              stop <- w477 stop-if-true
              n246 = Enqueue Element(queue=w478, element=w479, error in (no error)=w480) -> (error out=w477:errorcluster)  [unwired: 1 in, 2 out]
            }
          }
          frame Error {
            n247 = To Variant(anything=0) -> (Variant=w482:variant)
            n248 = Bundle("Command"="Exit", "Command class"="gen", "Variant"=w482) -> (w481:T7)  [unwired: 1 in]
            n249 = Enqueue Element(queue=w487, element=w481, error in (no error)=w486) -> ()  [unwired: 1 in, 3 out]
          }
        }
      }
      n250 = Bundle("command", "command class", variant) -> (w293:cluster{string, string, variant})  [unwired: 1 in]
      n251 = Bundle("command", "command class", variant) -> (w288:cluster{string, string, variant})  [unwired: 1 in]
      n252 = Bundle("command", "command class", variant) -> (w277:cluster{string, string, variant})  [unwired: 1 in]
      n253 = Obtain Queue(name (unnamed)="fastq", element data type=w293) -> (queue out=w256:refnum<queue>, error out=w259:errorcluster)  [unwired: 3 in, 1 out]
      n254 = Obtain Queue(name (unnamed)="medq", element data type=w288) -> (queue out=w260:refnum<queue>, error out=w257:errorcluster)  [unwired: 3 in, 1 out]
      n255 = Obtain Queue(name (unnamed)="slowq", element data type=w277) -> (queue out=w261:refnum<queue>, error out=w258:errorcluster)  [unwired: 3 in, 1 out]
      n256 = while {
        tunnel: w264 -> [w332]
        tunnel: w265 -> [w331]
        tunnel: [w330] -> w272
        tunnel: [w321] -> w274
        tunnel: w256 -> [w328]
        tunnel: w259 -> [w327]
        tunnel: w260 -> [w326]
        tunnel: w257 -> [w325]
        tunnel: w261 -> [w324]
        tunnel: w258 -> [w323]
        tunnel: w275 -> [w317]
        stop <- w320 stop-if-true
        # "DISTRIBUTOR\nAssigns 'mainq' commands to separate queues for each worker\n- operates on 1/16 slave timebase"
        n257 = Dequeue Element(queue=w332, error in (no error)=w331) -> (queue out=w330:refnum<queue>, element=w322:cluster{string, string, variant}, error out=w321:errorcluster)  [unwired: 1 in, 1 out]
        n258 = Unbundle(w322) -> (w329:string)  [unwired: 2 out]
        n259 = case shown="\"updui\"" w329 {
          tunnel: w328 -> [w335 _ _]
          tunnel: w327 -> [w334 _ _]
          tunnel: w326 -> [_ w337 _]
          tunnel: w325 -> [_ w336 _]
          tunnel: w324 -> [_ _ w340]
          tunnel: w323 -> [_ _ w339]
          tunnel: w322 -> [w333 w338 w341]
          frame "gen", Default {
            n260 = Enqueue Element(queue=w335, element=w333, error in (no error)=w334) -> ()  [unwired: 1 in, 3 out]
          }
          frame "instr" {
            n261 = Enqueue Element(queue=w337, element=w338, error in (no error)=w336) -> ()  [unwired: 1 in, 3 out]
          }
          frame "updui" {
            n262 = Enqueue Element(queue=w340, element=w341, error in (no error)=w339) -> ()  [unwired: 1 in, 3 out]
          }
        }
        n263 = Unbundle By Name(w321) -> ("status"=w320:bool)
        n264 = Scale By Power Of 2(n=-4, x=w317) -> (x*2^n=w318:dbl)
        n265 = Wait Until Next ms Multiple(millisecond multiple=w318) -> ()  [unwired: 1 out]
      }
      n266 = Release Queue(queue=w272, error in (no error)=w274) -> (error out=w271:errorcluster)  [unwired: 3 out]
      n267 = call <vilib>:"Simple Error Handler.vi"("error in (no error)"=w271) -> ()  [unwired: 1 in, 8 out]
      n268 = while {
        tunnel: [w434] -> w299
        tunnel: w259 -> [w429]
        tunnel: w256 -> [w430]
        tunnel: [w433] -> w298
        tunnel: w263 -> [w420]
        tunnel: w275 -> [w421]
        tunnel: w262 -> [w419]
        stop <- w418 stop-if-true
        # "Current command classes:\ngen,"
        # "WORKER I\nExecute upon 'mainq' commands: highest priority\n - operates on 1/8 slave timebase"
        n269 = Get Queue Status(queue=w430, error in (no error)=w429) -> (queue out=w433:refnum<queue>, error out=w434:errorcluster)  [unwired: 7 out]
        n270 = Dequeue Element(queue=w430, error in (no error)=w429) -> (queue out=w425:refnum<queue>, element=w424:cluster{string, string, variant}, error out=w432:errorcluster)  [unwired: 1 in, 1 out]
        n271 = Unbundle(w424) -> (w431:string, w427:string, w426:variant)
        n272 = case shown="\"gen\"" w427 {
          tunnel: w432 -> [w440 w458]
          tunnel: w431 -> [w437 _]
          tunnel: [w439 FALSE] -> _
          tunnel: [w438 ""] -> w428
          tunnel: w426 -> [_ _]
          tunnel: w425 -> [_ w460]
          tunnel: w424 -> [_ w459]
          tunnel: w420 -> [w435 _]
          tunnel: w419 -> [w436 _]
          frame "gen" {
            n273 = case shown="\"Exit\"" w437 {
              tunnel: w440 -> [_ _ _ _]
              tunnel: [FALSE FALSE TRUE FALSE] -> w439
              tunnel: ["" "Stopping..." "Closing down..." "Initializing interface..."] -> w438
              tunnel: w436 -> [_ _ _ w449]
              tunnel: w435 -> [_ _ _ w451]
              frame Default {
              }
              frame "BeginStop" {
              }
              frame "Exit" {
              }
              frame "Init" {
                n274 = call "UIinitializationCommands.vi"() -> ("array of cmds"=w453:T11)  [unwired: 2 in]
                n275 = Unbundle(w449) -> (w448:T4, w447:cluster{string, "qintoMain":refnum<user-event>})
                n276 = call "changeLED_event.vi"("eventcluster"=w448, "LED?"="GUI-busy", "newStatus"=TRUE, "ctlarr"=w451) -> ()  [unwired: 9 in, 3 out]
                n277 = call "enqMulti.vi"("array of cmds"=w453, "eventcluster"=w447) -> ()  [unwired: 9 in, 1 out]
              }
            }
          }
          frame Default {
            n278 = Enqueue Element(queue=w460, element=w459, error in (no error)=w458) -> ()  [unwired: 1 in, 3 out]
          }
        }
        n279 = Unbundle By Name(w434) -> ("status"=w418:bool)
        n280 = Scale By Power Of 2(n=-3, x=w421) -> (x*2^n=w422:dbl)
        n281 = Wait Until Next ms Multiple(millisecond multiple=w422) -> ()  [unwired: 1 out]
        n282 = call "writeNotification.vi"("string"=w428, "Array"=w420) -> ()  [unwired: 10 in]
      }
      n283 = while {
        tunnel: [w407] -> w284
        tunnel: w257 -> [w403]
        tunnel: w260 -> [w404]
        tunnel: w263 -> [w392]
        tunnel: w275 -> [w394]
        tunnel: [w393] -> w285
        tunnel: w262 -> [w391]
        stop <- w395 stop-if-true
        # "Current command classes:\ninstr,"
        # "WORKER II\nExecute upon 'mainq' commands: medium priority\n - operates on 1/4 slave timebase"
        n284 = Get Queue Status(queue=w404, error in (no error)=w403) -> (queue out=w393:refnum<queue>, error out=w407:errorcluster)  [unwired: 7 out]
        n285 = Dequeue Element(queue=w404, error in (no error)=w403) -> (queue out=w399:refnum<queue>, element=w398:cluster{string, string, variant}, error out=w406:errorcluster)  [unwired: 1 in, 1 out]
        n286 = Unbundle(w398) -> (w405:string, w401:string, w400:variant)
        n287 = case shown="\"instr\"" w401 {
          tunnel: w406 -> [w412 w415]
          tunnel: w405 -> [w410 _]
          tunnel: [w411 ""] -> w402
          tunnel: w400 -> [w408 _]
          tunnel: w399 -> [_ w417]
          tunnel: w398 -> [_ w416]
          tunnel: w392 -> [w409 _]
          tunnel: w391 -> [_ _]
          frame "instr" {
            n288 = case shown="Default" w410 {
              tunnel: w412 -> [_ _]
              tunnel: ["" _] -> w411
              tunnel: w409 -> [_ _]
              tunnel: w408 -> [_ _]
              frame Default {
              }
              frame "initLIA" {
              }
            }
          }
          frame Default {
            n289 = Enqueue Element(queue=w417, element=w416, error in (no error)=w415) -> ()  [unwired: 1 in, 3 out]
          }
        }
        n290 = Unbundle By Name(w407) -> ("status"=w395:bool)
        n291 = Scale By Power Of 2(n=-2, x=w394) -> (x*2^n=w396:dbl)
        n292 = call "writeNotification.vi"("string"=w402, "Array"=w392) -> ()  [unwired: 10 in]
        n293 = Wait Until Next ms Multiple(millisecond multiple=w396) -> ()  [unwired: 1 out]
      }
      n294 = while {
        tunnel: [w358] -> w281
        tunnel: w258 -> [w354]
        tunnel: w261 -> [w355]
        tunnel: w263 -> [w343]
        tunnel: w275 -> [w345]
        tunnel: [w344] -> w282
        tunnel: w262 -> [w342]
        stop <- w346 stop-if-true
        # "Current command classes:\nupdui, disb"
        # "WORKER III\nExecute upon 'mainq' commands: low priority\n - operates on slave timebase"
        n295 = Get Queue Status(queue=w355, error in (no error)=w354) -> (queue out=w344:refnum<queue>, error out=w358:errorcluster)  [unwired: 7 out]
        n296 = Dequeue Element(queue=w355, error in (no error)=w354) -> (queue out=w350:refnum<queue>, element=w349:cluster{string, string, variant}, error out=w357:errorcluster)  [unwired: 1 in, 1 out]
        n297 = Unbundle(w349) -> (w356:string, w352:string, w351:variant)
        n298 = case shown="\"updui\"" w352 {
          tunnel: w357 -> [w364 w385 w388]
          tunnel: w356 -> [w362 w383 _]
          tunnel: [w363 w384 ""] -> w353
          tunnel: w351 -> [w360 _ _]
          tunnel: w350 -> [_ _ w390]
          tunnel: w349 -> [_ _ w389]
          tunnel: w343 -> [w361 _ _]
          tunnel: w342 -> [w359 _ _]
          frame "updui" {
            n299 = case shown="\"InitFin\"" w362 {
              tunnel: w364 -> [_ _ _ _ _ _]
              tunnel: ["" w366 "Notifications cleared." "Interface initialization complete." _ _] -> w363
              tunnel: w361 -> [_ w368 _ w374 w378 w381]
              tunnel: w360 -> [_ w367 _ _ w379 w382]
              tunnel: w359 -> [_ _ _ w373 _ _]
              frame Default {
              }
              frame "setPowerLim" {
                n300 = call "setPowerLim.vi"("ctlref"=w368, "Variant"=w367) -> ("notification"=w366:string)
              }
              frame "clearNotifications" {
                n301 = control-ref of="Notifications"() -> (w371:refnum<vi>)
                n302 = property class="Str"(reference=w371, "Value"="") -> ()  [unwired: 1 in, 2 out]
              }
              frame "InitFin" {
                n303 = Unbundle(w373) -> (w372:T4)  [unwired: 1 out]
                n304 = call "changeLED_event.vi"("eventcluster"=w372, "LED?"="GUI-busy", "newStatus"=FALSE, "ctlarr"=w374) -> ()  [unwired: 9 in, 3 out]
              }
              frame "toggleInstrSett" {
                n305 = call "toggleCtlVis.vi"("ctlarr"=w378, "Variant"=w379) -> ()  [unwired: 8 in, 2 out]
              }
              frame "toggleVISAfields" {
                n306 = call "toggleCtlVis.vi"("ctlarr"=w381, "Variant"=w382, "tag?"="visa") -> ()  [unwired: 7 in, 2 out]
              }
            }
          }
          frame "disb" {
            n307 = case shown="\"enableInstrSett\"" w383 {
              tunnel: w385 -> [_ _]
              tunnel: ["" _] -> w384
              frame Default {
              }
              frame "enableInstrSett" {
              }
            }
          }
          frame Default {
            n308 = Enqueue Element(queue=w390, element=w389, error in (no error)=w388) -> ()  [unwired: 1 in, 3 out]
          }
        }
        n309 = Unbundle By Name(w358) -> ("status"=w346:bool)
        n310 = Scale By Power Of 2(n=0, x=w345) -> (x*2^n=w347:dbl)
        n311 = call "writeNotification.vi"("string"=w353, "Array"=w343) -> ()  [unwired: 10 in]
        n312 = Wait Until Next ms Multiple(millisecond multiple=w347) -> ()  [unwired: 1 out]
      }
      n313 = Unregister For Events(event registration refnum=w297, error in=w270) -> (error out=w267:errorcluster)
      n314 = case shown="True" FALSE {
        tunnel: w262 -> [_ w306]
        tunnel: [w301 w305] -> w268
        tunnel: w267 -> [w301 _]
        frame False {
        }
        frame True {
          n315 = Unbundle(w306) -> (w304:T4, w303:cluster{string, "qintoMain":refnum<user-event>})
          n316 = for {
            N: 2 -> [_]
            tunnel: [w309] -> w305
            tunnel: w304 -> [w308]
            tunnel: w303 -> [w307]
            i -> [w310]
            n317 = case shown="1" w310 {
              tunnel: [w313 w316] -> w309
              tunnel: w308 -> [w312 _]
              tunnel: w307 -> [_ w314]
              frame 0, Default {
                n318 = Unbundle(w312) -> ("chgStatusLED"=w311:refnum<user-event>)  [unwired: 1 out]
                n319 = Destroy User Event(user event=w311) -> (error out=w313:errorcluster)  [unwired: 1 in]
              }
              frame 1 {
                n320 = Unbundle(w314) -> ("qintoMain"=w315:refnum<user-event>)  [unwired: 1 out]
                n321 = Destroy User Event(user event=w315) -> (error out=w316:errorcluster)  [unwired: 1 in]
              }
            }
          }
        }
      }
      n322 = call <vilib>:"Simple Error Handler.vi"("error in (no error)"=w268) -> ()  [unwired: 4 in, 5 out]
      n323 = Release Queue(queue=w298, error in (no error)=w299) -> (error out=w300:errorcluster)  [unwired: 3 out]
      n324 = Release Queue(queue=w285, error in (no error)=w284) -> (error out=w286:errorcluster)  [unwired: 3 out]
      n325 = Release Queue(queue=w282, error in (no error)=w281) -> (error out=w283:errorcluster)  [unwired: 3 out]
      n326 = call <vilib>:"Simple Error Handler.vi"("error in (no error)"=w300) -> ()  [unwired: 1 in, 8 out]
      n327 = call <vilib>:"Simple Error Handler.vi"("error in (no error)"=w286) -> ()  [unwired: 1 in, 8 out]
      n328 = call <vilib>:"Simple Error Handler.vi"("error in (no error)"=w283) -> ()  [unwired: 1 in, 8 out]
    }
  }
